vi "Find Vector Distance.vi"(1 "Point B":T1, 2 "Point A":T1) -> (0 "Distance Between A and B":dbl)   [LabVIEW 2018]
uses:
  Classes/Video Cam Processor/Private/Hull Point STYP.ctl
  c7a169ae-5fa5-4041-bcc8-af80f43c5b70.vi
  Classes/Video Cam Processor/Video Cam Processor.lvclass
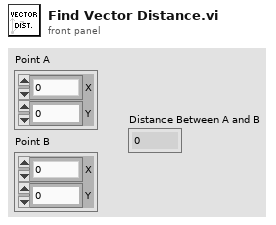
[diagram p1: front panel]
types:
  T1 = typedef "Video Cam Processor.lvclass/Hull Point STYP.ctl" = cluster{"X":i32, "Y":i32}
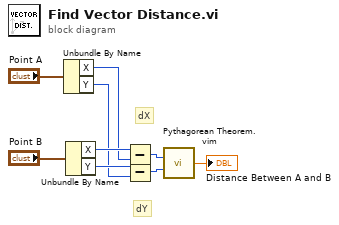
[diagram p0: block diagram]
diagram:
  # "dY"
  # "dX"
  n1 = Unbundle By Name("Point A") -> ("X"=w6:i32, "Y"=w4:i32)
  n2 = Unbundle By Name("Point B") -> ("X"=w7:i32, "Y"=w5:i32)
  n3 = Subtract(x=w7, y=w6) -> (x-y=w3:i32)
  n4 = Subtract(x=w5, y=w4) -> (x-y=w2:i32)
  n5 = call "Pythagorean Theorem.vim"("X"=w3, "Y"=w2) -> ("Z"=→"Distance Between A and B":dbl)  [unwired: 13 in]
